vi "DestructSDK.vi"   [LabVIEW 2010]
uses:
  Program Files/Meadowlark Optics/Blink 1920 HDMI/SDK/Blink_C_wrapper.dll
panel:
  # "Call this function when you are done using LabVIEW\nIn order to properly shut down the lower level code \nthis function will force LabVIEW to exit"
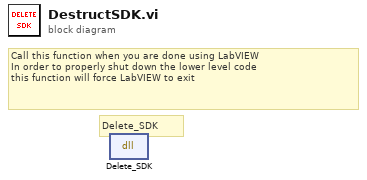
[diagram p0: block diagram]
diagram:
  # "Call this function when you are done using LabVIEW\nIn order to properly shut down the lower level code \nthis function will force LabVIEW to exit"
  # "Delete_SDK"
  n1 = dll-call lib="C:/Program Files/Meadowlark Optics/Blink 1920 HDMI/SDK/Blink_C_wrapper.dll" fn="Delete_SDK"() -> ()  [unwired: 4 in, 2 out]
